vi "Get ADAS Replay HIL Installed Info.vi"() -> (3 "ADAS Replay HIL pkg info":string)   [LabVIEW 2023, in "Plugin Generator.lvlib"]
uses:
  Plugin Generator.lvlib
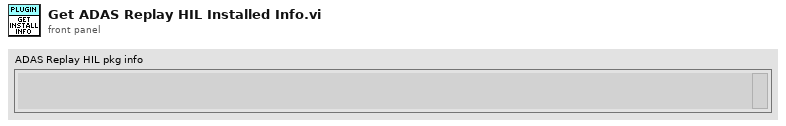
[diagram p1: front panel]
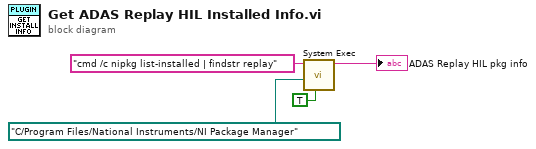
[diagram p0: block diagram]
diagram:
  n1 = call <vilib>:"System Exec.vi"("run minimized? (F)"=TRUE, "working directory"=path "C:/Program Files/National Instruments/NI Package Manager", "command line"="cmd /c nipkg list-installed | findstr replay") -> ("standard output"=→"ADAS Replay HIL pkg info":string)  [unwired: 5 in, 3 out]
